vi "Run Service.vi"(11 "server settings":T1) -> (0 "error out":errorcluster)   [LabVIEW 2021, in "MeasurementServerTests.lvlib" / "Measurement Service Tests.lvlib" / "Continuous Counting Measurement2.lvclass"]
uses:
  Continuous Counting Measurement2.lvclass
  Runtime/Measurements/Helpers/TypeDefs/Measurement Server User Settings.ctl
  Runtime/Measurements/Helpers/TypeDefs/Stop Server User Event.ctl
  Runtime/Measurements/Helpers/TypeDefs/Measurement Service Version.ctl
  C:/Dev/github/ni/measurementlink-labview/Source/Runtime/Measurements/Measurement Plugin Service/Measurement Plugin Service.lvclass
  Runtime/Measurements/NI Measurement Plug-In SDK.lvlib
panel:
  # "Run this VI to start the measurement service.  A window will appear that provides basic information about the running service.\n\nUse the stop button on the window that appears to stop the measurement service."
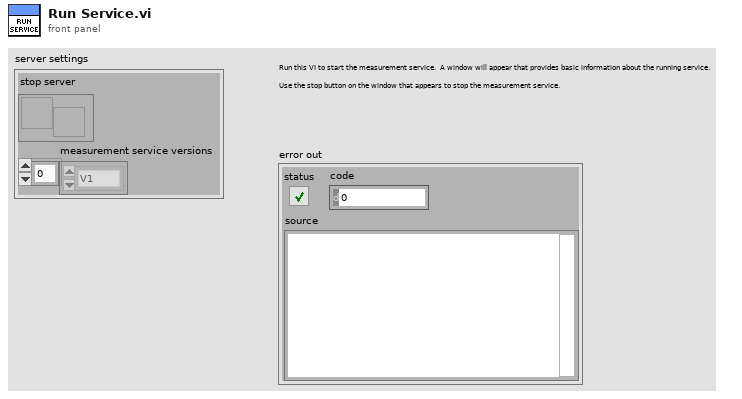
[diagram p1: front panel]
types:
  T1 = typedef "NI Measurement Plug-In SDK.lvlib/Measurement Server User Settings.ctl" = cluster{"stop server":T2, "measurement service versions":T3[]}
  T2 = typedef "NI Measurement Plug-In SDK.lvlib/Stop Server User Event.ctl" = refnum<user-event>
  T3 = typedef "NI Measurement Plug-In SDK.lvlib/Measurement Service Version.ctl" = enum16{"V1", "V2"}
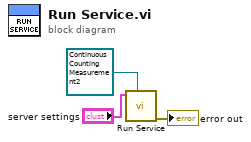
[diagram p0: block diagram]
diagram:
  n1 = call "Run Service.vi"("measurement"=refnum<class "Continuous Counting Measurement2.lvclass"> refnum ("MeasurementServerTests.lvlib:Measurement Service Tests.lvlib:Continuous Counting Mesurement2.lvclass"), "measurementlink server user settings"="server settings") -> ("error out"=→"error out":errorcluster)  [unwired: 9 in]
